vi "Learn fiducial.vi"(2 "template path":path=path "C:/Users/HEP/Documents/Aerotech gantry/Sindhu/Pattern recog/fidcloseSq.png") -> (1 "Template":T1(plugin-control))   [LabVIEW 2020]
uses:
  <vilib>/vision/NI_Vision_Development_Module.lvlib
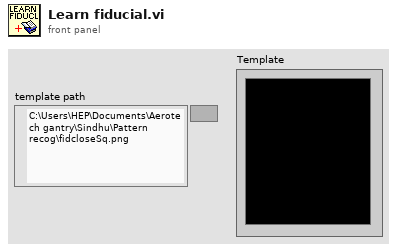
[diagram p1: front panel]
types:
  T1 = typedef "IMAQ Image.ctl" = refnum<image>
  T2 = typedef "Image Type" = u32
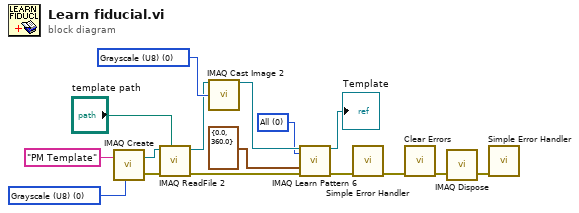
[diagram p0: block diagram]
diagram:
  w2 = 0 items=["All", "Low Discrepancy Sampling", "Grayscale Value Pyramid", "Gradients Pyramid"] ("Algorithm")
  w12 = T2 0 items=["Grayscale (U8)", "Grayscale (I16)", "Grayscale (SGL)", "Complex (CSG)", "RGB (U32)", "HSL (U32)", "RGB (U64)", "Grayscale (U16)"] ("Image Type")
  w15 = T2 0 items=["Grayscale (U8)", "Grayscale (I16)", "Grayscale (SGL)", "Complex (CSG)", "RGB (U32)", "HSL (U32)", "RGB (U64)", "Grayscale (U16)"] ("Image Type")
  n1 = call "IMAQ Create"("Image Name"="PM Template", "Image Type"=w15) -> ("New Image"=w13:T1, "error out"=w14:errorcluster)  [unwired: 3 in]
  n2 = call "IMAQ ReadFile 2"("File Path"="template path", "error in (no error)"=w14, "Image"=w13) -> ("error out"=w7:errorcluster, "Image Out"=w11:T1)  [unwired: 4 in, 3 out]
  n3 = call "IMAQ Cast Image 2"("Image Src"=w11, "Image Type"=w12) -> ("Image Dst Out"=w4:T1)  [unwired: 12 in, 1 out]
  n4 = call "IMAQ Learn Pattern 6"("Image"=w4, "Algorithm"=w2, "Angle Range"=cluster{"Start Angle":sgl, "End Angle":sgl} {"Start Angle"=0.0, "End Angle"=360.0}, "error in (no error)"=w7) -> ("Template Image Out"=→"Template":T1, "error out"=w9:errorcluster)  [unwired: 9 in, 1 out]
  n5 = call <vilib>:"Simple Error Handler.vi"("error in (no error)"=w9) -> ("error out"=w10:errorcluster)  [unwired: 4 in, 4 out]
  n6 = call <vilib>:"Clear Errors.vi"("error in (no error)"=w10) -> ("error out"=w6:errorcluster)  [unwired: 5 in, 1 out]
  n7 = call "IMAQ Dispose"("error in (no error)"=w6) -> ("error out"=w5:errorcluster)  [unwired: 5 in]
  n8 = call <vilib>:"Simple Error Handler.vi"("error in (no error)"=w5) -> ()  [unwired: 4 in, 5 out]
